vi "Configure DC Current Filter.vi"(8 "error in (no error)":errorcluster, 10 "Enable DC Current Filter (Disable)":bool, 11 "VISA resource name":refnum<visa-resource-name>) -> (0 "error out":errorcluster, 3 "VISA resource name out":refnum<visa-resource-name>)   [LabVIEW 2020, in "Library Instrument & Equipement.lvlib" / "Library Multimeter.lvlib" / "RIGOL DM3058.lvlib"]
doc: "Configures the DC Current Filter. \n\n<B>Note:</B>\nThis VI only applies to RIGOL DM3058 model."
uses:
  RIGOL DM3058.lvlib
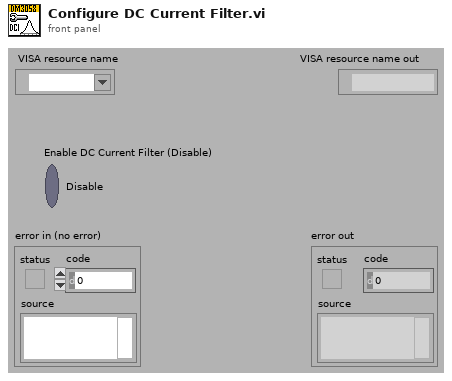
[diagram p1: front panel]
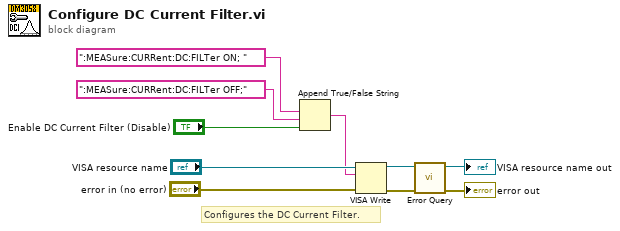
[diagram p0: block diagram]
diagram:
  # "Configures the DC Current Filter."
  n1 = Append True/False String(1:"Enable DC Current Filter (Disable)", 2:":MEASure:CURRent:DC:FILTer OFF;", 3:":MEASure:CURRent:DC:FILTer ON; ") -> (0:w6:string)  [unwired: 1 out]
  n2 = VISA Write(VISA resource name="VISA resource name", write buffer=w6, error in (no error)="error in (no error)") -> (VISA resource name out=w4:refnum<visa-resource-name>, error out=w3:errorcluster)  [unwired: 1 out]
  n3 = call "Error Query.vi"("error in (no error)"=w3, "VISA resource name"=w4) -> ("error out"=→"error out":errorcluster, "VISA resource name out"=→"VISA resource name out":refnum<visa-resource-name>)  [unwired: 6 in, 2 out]
